vi "Window-8-bit Export Codec.vi"() -> (0 "error out (no error)":errorcluster)   [LabVIEW 2020]
uses:
  Typedefs/Save-Load enum.ctl
  Global Variables/General Globals.vi
panel:
  in  "Codec Selector":u16(ring) items=["Intel IYUV codec", "Cinepak Codec by Radius", "Microsoft Video 1", "FF Video Codec 1 (FFV1) (NI Vision)", "Motion JPEG (NI Vision)", "Y800 Uncompressed Grey Scale (NI Vision)", "YUV 4:2:0 Planar (NI Vision)"]
  in  "Cancel":bool
  in  "OK":bool
  # "Choose a compression codec. Codecs are compression decoders each offering different image quality and file compression characteristics."
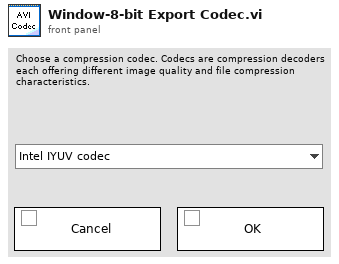
[diagram p1: front panel]
types:
  T1 = typedef "Save-Load enum.ctl" = enum16{"Save to file", "Load from file", "Compare from file", "Save Backup"}
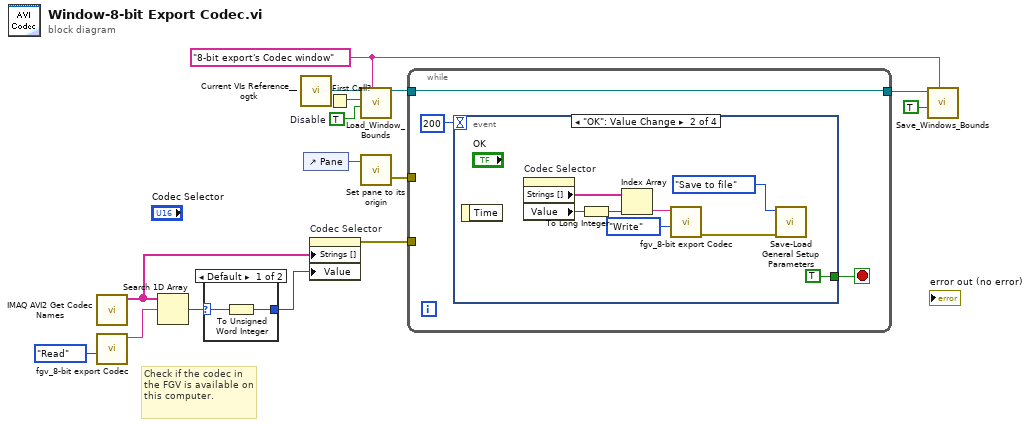
[diagram p0: block diagram]
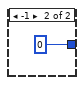
[diagram p2: hidden frame]
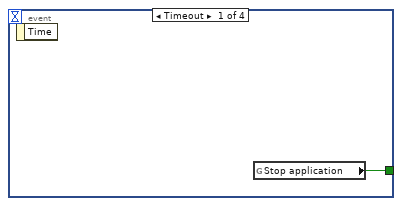
[diagram p3: hidden frame]
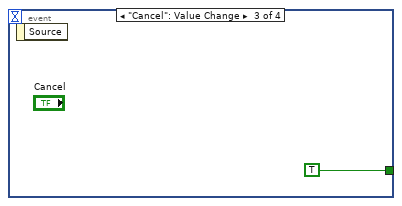
[diagram p4: hidden frame]
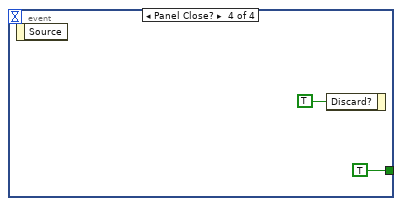
[diagram p5: hidden frame]
diagram:
  w11 = TRUE  # Disable
  w10 = "8-bit export's Codec window" ("Window Name (i.e. Key)")
  # "Check if the codec in the FGV is available on this computer."
  n1 = call "IMAQ AVI2 Get Codec Names"() -> ("Codec Names"=w3:string[])  [unwired: 10 in, 1 out]
  n2 = call "fgv_8-bit export Codec.vi"("Function"=enum16{"Intialize", "Write", "Read", "Clear"}."Read") -> ("AVI mode"=w5:string)  [unwired: 9 in, 1 out]
  n3 = Search 1D Array(1D array=w3, element=w5) -> (index of element=w4:i32)  [unwired: 1 in]
  n4 = case shown="Default" w4 {
    selector: w4 -> [w17 _]
    tunnel: [w16 u16 0 ("index of element")] -> w2
    frame Default {
      n5 = To Unsigned Word Integer(number=w17) -> (unsigned 16bit integer=w16:u16)
    }
    frame -1 {
    }
  }
  n6 = call <userlib>:"Current VIs Reference__ogtk.vi"() -> ("Current VI's reference"=w13:refnum<vi>)  [unwired: 5 in]
  n7 = control-ref of="Pane"() -> (w15:refnum<vi>)
  n8 = property on="Codec Selector" class="Ring (strict)"("Strings []"=w3, "Value"=w2) -> (error out=w1:errorcluster)  [unwired: 2 in, 1 out]
  n9 = First Call?() -> (First Call?: T/F=w12:bool)
  n10 = call "Load_Window_Bounds.vi"("Window Name (i.e. Key)"=w10, "Disable"=w11, "First Call"=w12, "Window VI's Ref"=w13) -> ("reference out"=w7:refnum<vi>)  [unwired: 4 in, 3 out]
  n11 = call <userlib>:"Set pane to its origin.vi"("Pane Reference"=w15) -> ("error out (no error)"=w14:errorcluster)  [unwired: 9 in, 1 out]
  n12 = while {
    tunnel: w14 -> [_]
    tunnel: w7 -> [w20]
    tunnel: [w20] -> w8
    tunnel: w1 -> [_]
    stop <- w21 stop-if-true
    n13 = event shown="[1] \"OK\": Value Change" {
      selector: _ -> [_ _ _ _]
      dyn-events: _ -> [_ _ _ _]
      timeout: 200 -> [_ _ _ _]
      tunnel: [w22 TRUE TRUE TRUE] -> w21
      event Timeout {
        n14 = event-data() -> ()  [unwired: 1 in, 1 out]
        n15 = global read "General Globals.vi" "Stop application"() -> (w22:bool)
      }
      event "OK": Value Change {
        n16 = event-data() -> ()  [unwired: 1 in, 1 out]
        n17 = property on="Codec Selector" class="Ring (strict)"() -> ("Strings []"=w27:string[], "Value"=w28:u16)  [unwired: 2 in, 2 out]
        n18 = To Long Integer(number=w28) -> (32bit integer=w29:i32)
        n19 = Index Array(array=w27, index=w29) -> (element=w25:string)
        n20 = call "fgv_8-bit export Codec.vi"("Function"=enum16{"Intialize", "Write", "Read", "Clear"}."Write", "Codec"=w25) -> ("error out"=w24:errorcluster)  [unwired: 8 in, 1 out]
        n21 = call "Save-Load General Setup Parameters.vi"("error in"=w24, "Function"=Save-Load_enum."Save to file") -> ()  [unwired: 9 in, 1 out]
      }
      event "Cancel": Value Change {
        n22 = event-data() -> ()  [unwired: 1 in, 1 out]
      }
      event Panel Close? {
        n23 = event-data() -> ()  [unwired: 1 in, 1 out]
        n24 = event-data("Discard?"=TRUE) -> ()  [unwired: 1 in, 1 out]
      }
    }
  }
  n25 = call "Save_Windows_Bounds.vi"("Window Name (i.e. Key)"=w10, "Front Panel Window:Open"=TRUE, "Window VI's Ref"=w8) -> ()  [unwired: 8 in, 1 out]
